vi "Bootloader.vi"() -> ()   [LabVIEW 2010]
uses:
  <vilib>/Utility/sysdir.llb/System Directory Type.ctl
  <vilib>/Instr/_visa.llb/VISA Configure Serial Port (Instr).vi
panel:
  in  "start path":path=path "<Not A Path>"
  in  "Run 3":bool
  in  "Run 2":bool
  in  "Exit":bool
  in  "Run":bool
  in  "Resource name:":refnum<visa-resource-name>
  in  "Path to firmware file (.hex):":path
  # "Caution: Make sure the right Firmware file is selected before Update the Harp device. Selecting\na Firmware that was not designed for the target Harp device may cause permanent damage."
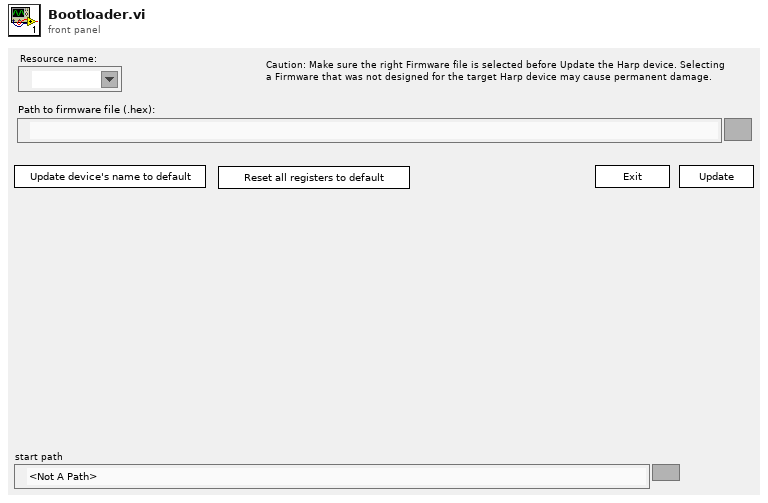
[diagram p1: front panel]
types:
  T1 = typedef "System Directory Type.ctl" = i32
  T2 = cluster{"reg. address":u8, "address content (en)":u8, "address content (dis)":u8, "fw .hex file path":path, "updater path":path}
  T3 = cluster{"reg. address":u8, "address content (en)":u8, "address content (dis)":u8, "Has .X":bool}[]
  T4 = cluster{"reg. address":u8, "address content (en)":u8, "address content (dis)":u8, "Has .X":bool}
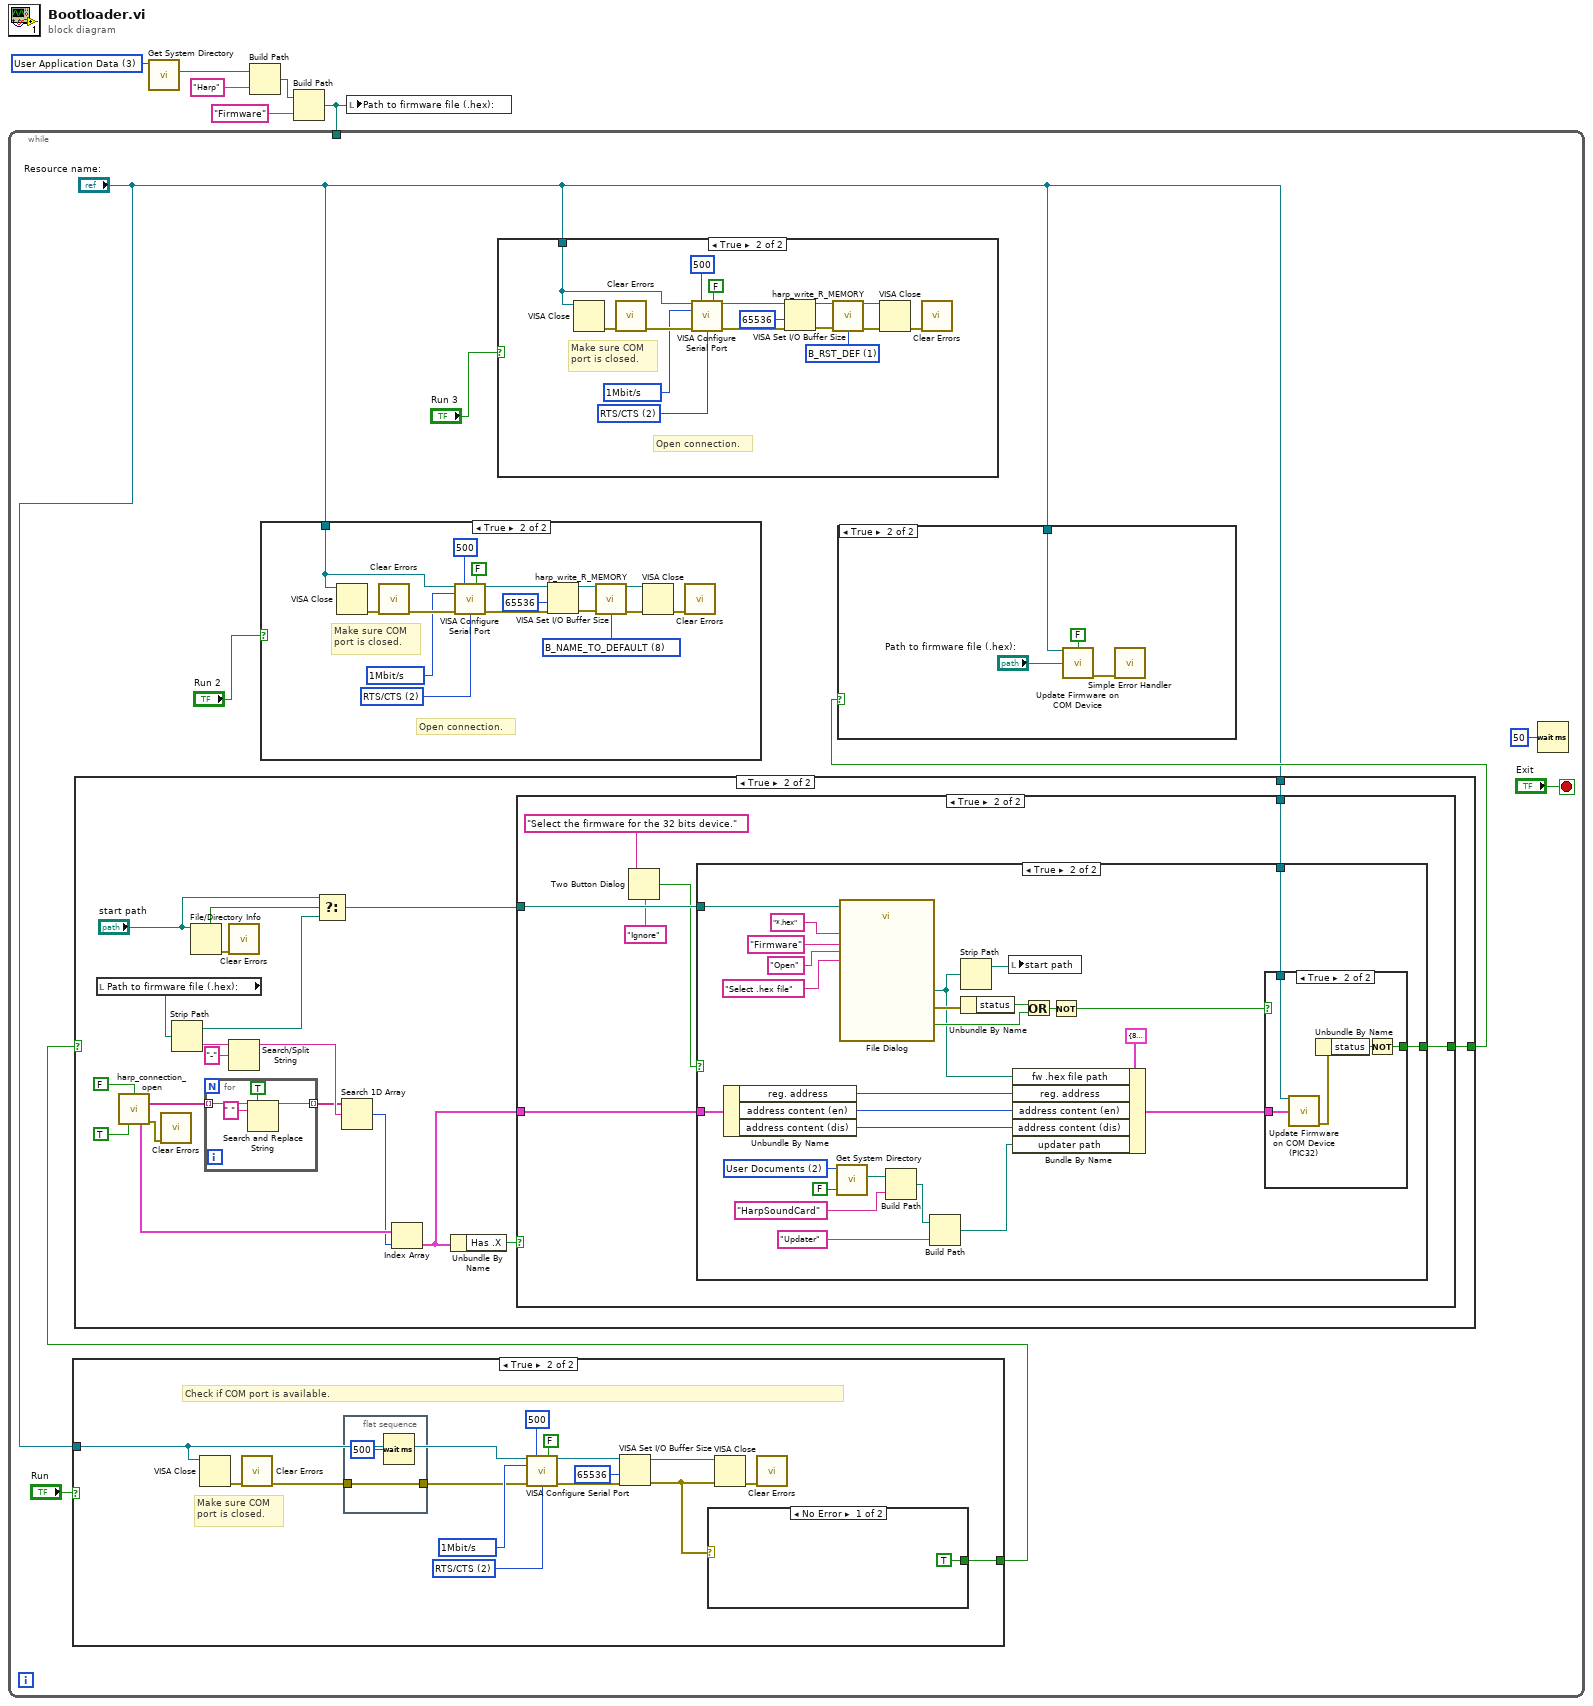
[diagram p0: block diagram]
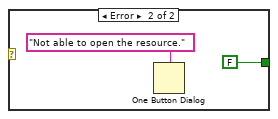
[diagram p3: hidden frame]
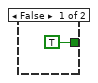
[diagram p5: hidden frame]
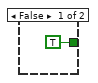
[diagram p6: hidden frame]
diagram:
  w4 = T1 3 items=["User Home"=0, "User Desktop"=1, "User Documents"=2, "User Application Data"=3, "User Preferences"=4, "User Temporary"=5, "Public Documents"=6, "Public Application Data"=7, "Public Preferences"=8, "Public Cache"=13, "System Core Libraries"=9, "System Installed Libraries"=10, "Application Files"=11, "Boot Volume Root"=12] ("system directory type")
  n1 = call <vilib>:"Get System Directory.vi"("system directory type"=w4) -> ("system directory"=w5:path)  [unwired: 10 in]
  n2 = Build Path(base path=w5, name or relative path="Harp") -> (appended path=w2:path)
  n3 = Build Path(base path=w2, name or relative path="Firmware") -> (appended path=w1:path)
  n4 = while {
    tunnel: w1 -> [_]
    stop <- "Exit" stop-if-true
    n5 = case shown="True" "Run" {
      selector: "Run" -> [w15 _]
      tunnel: "Resource name:" -> [_ w21]
      tunnel: [w15 w16] -> w7
      frame False {
      }
      frame True {
        w26 = u32 1000000 items=["250Kbit/s"=250000, "500kbit/s"=500000, "1Mbit/s"=1000000, "2Mbit/s"=2000000, "4Mbit/s"=4000000] ("baud rate")
        w27 = u16 2 items=["None", "XON/XOFF", "RTS/CTS", "XON/XOFF & RTS/CTS", "DTR/DSR", "XON/XOFF & DTR/DSR"] ("flow control (0:none)")
        # "Check if COM port is available."
        # "Make sure COM\nport is closed."
        n6 = VISA Close(VISA resource name=w21) -> (error out=w30:errorcluster)  [unwired: 1 in]
        n7 = call <vilib>:"Clear Errors.vi"("error in (no error)"=w30) -> ("error out"=w19:errorcluster)  [unwired: 6 in]
        n8 = flat-sequence {
          tunnel: w19 -> [w35]
          tunnel: [w35] -> w18
          frame #0 {
            n9 = Wait (ms)(milliseconds to wait=u32 500) -> ()  [unwired: 1 out]
          }
        }
        n10 = call-poly "VISA Configure Serial Port"("VISA resource name"=w21, "timeout (10sec)"=u32 500, "Enable Termination\nChar (T)"=FALSE ("Enable Termination\nChar (T)"), "baud rate (9600)"=w26, "error in (no error)"=w18, "flow control (0:none)"=w27) -> ("VISA resource name out"=w23:refnum<visa-resource-name>, "error out"=w24:errorcluster)  [unwired: 8 in]
        n11 = VISA Set I/O Buffer Size(VISA resource name=w23, size (4096)=u32 65536, error in (no error)=w24) -> (VISA resource name out=w20:refnum<visa-resource-name>, error out=w17:errorcluster)  [unwired: 1 in]
        n12 = case shown="No Error" w17 {
          tunnel: [TRUE FALSE] -> w16
          frame No Error {
          }
          frame Error {
            n13 = One Button Dialog(message="Not able to open the resource.") -> ()  [unwired: 1 in, 1 out]
          }
        }
        n14 = VISA Close(VISA resource name=w20, error in (no error)=w17) -> (error out=w22:errorcluster)
        n15 = call <vilib>:"Clear Errors.vi"("error in (no error)"=w22) -> ()  [unwired: 6 in, 1 out]
      }
    }
    n16 = case shown="True" w7 {
      selector: w7 -> [w36 _]
      tunnel: "Resource name:" -> [_ w40]
      tunnel: [w36 w39] -> w10
      frame False {
      }
      frame True {
        n17 = local read "Path to firmware file (.hex):"() -> (w44:path)
        n18 = call "harp_connection_open.vi"("launch dialog"=FALSE, "get lists only"=TRUE) -> ("Devices Name List"=w41:string[], "Devices X. settings"=w50:T3, "error out"=w42:errorcluster)  [unwired: 8 in, 3 out]
        n19 = call <vilib>:"Clear Errors.vi"("error in (no error)"=w42) -> ()  [unwired: 6 in, 1 out]
        n20 = Strip Path(path=w44) -> (stripped path=w54:path, name=w45:string)
        n21 = File/Directory Info(path="start path") -> (directory=w52:bool, error out=w37:errorcluster)  [unwired: 1 in, 5 out]
        n22 = for {
          tunnel: w41 -> [w101] mode=indexing
          tunnel: [w102] -> w47 mode=indexing
          n23 = Search and Replace String(replace all?=TRUE ("replace all? (F)"), input string=w101, search string=" ") -> (result string=w102:string)  [unwired: 5 in, 3 out]
        }
        n24 = call <vilib>:"Clear Errors.vi"("error in (no error)"=w37) -> ()  [unwired: 6 in, 1 out]
        n25 = Search/Split String(string=w45, search string/char (-)="-") -> (substring before match=w48:string)  [unwired: 1 in, 2 out]
        n26 = Select(t="start path", s=w52, f=w54) -> (s? t:f=w55:path)
        n27 = Search 1D Array(1D array=w47, element=w48) -> (index of element=w49:i32)  [unwired: 1 in]
        n28 = Index Array(array=w50, index=w49) -> (element=w51:T4)
        n29 = Unbundle By Name(w51) -> ("Has .X"=w56:bool)
        n30 = case shown="True" w56 {
          tunnel: w51 -> [_ w64]
          tunnel: w55 -> [_ w63]
          tunnel: w40 -> [_ w61]
          tunnel: [TRUE ("get lists only") w60] -> w39
          frame False {
          }
          frame True {
            n31 = Two Button Dialog(message="Select the firmware for the 32 bits device.", 1:"Ignore" ("F button name (\"Cancel\")")) -> (T button?=w58:bool)  [unwired: 1 in]
            n32 = case shown="True" w58 {
              tunnel: w64 -> [_ w92]
              tunnel: w63 -> [_ w91]
              tunnel: w61 -> [_ w90]
              tunnel: [TRUE w89] -> w60
              frame False {
              }
              frame True {
                w69 = T1 2 items=["User Home"=0, "User Desktop"=1, "User Documents"=2, "User Application Data"=3, "User Preferences"=4, "User Temporary"=5, "Public Documents"=6, "Public Application Data"=7, "Public Preferences"=8, "Public Cache"=13, "System Core Libraries"=9, "System Installed Libraries"=10, "Application Files"=11, "Boot Volume Root"=12] ("system directory type")
                n33 = Unbundle By Name(w92) -> ("reg. address"=w85:u8, "address content (en)"=w86:u8, "address content (dis)"=w87:u8)
                n34 = call <vilib>:"Get System Directory.vi"("create directory if not found? (F)"=FALSE, "system directory type"=w69) -> ("system directory"=w71:path)  [unwired: 9 in]
                n35 = call "File Dialog"("start path"=w91, "prompt"="Select .hex file" ("button label"), "button label"="Open", "pattern (all files)"="*.hex", "pattern label"="Firmware" ("button label")) -> ("selected path"=w76:path, "cancelled"=w77:bool, "error out"=w79:errorcluster)  [unwired: 7 in, 1 out]
                n36 = Build Path(base path=w71, name or relative path="HarpSoundCard") -> (appended path=w73:path)
                n37 = Build Path(base path=w73, name or relative path="Updater") -> (appended path=w68:path)
                n38 = Strip Path(path=w76) -> (stripped path=w80:path)  [unwired: 1 out]
                n39 = Unbundle By Name(w79) -> ("status"=w78:bool)
                n40 = local write "start path"(w80) -> ()
                n41 = Bundle By Name(cluster=T2 {"reg. address"=82, "address content (en)"=82, "address content (dis)"=82, "fw .hex file path"=path "Fir", "updater path"=path "Fir"} (".X settings"), "fw .hex file path"=w76, "reg. address"=w85, "address content (en)"=w86, "address content (dis)"=w87, "updater path"=w68) -> (w75:T2)
                n42 = Or(x=w78, y=w77) -> (x .or. y?=w67:bool)
                n43 = Not(x=w67) -> (.not. x?=w66:bool)
                n44 = case shown="True" w66 {
                  selector: w66 -> [w93 _]
                  tunnel: w75 -> [_ w98]
                  tunnel: w90 -> [_ w97]
                  tunnel: [w93 w94] -> w89
                  frame False {
                  }
                  frame True {
                    n45 = call "Update Firmware on COM Device (PIC32).vi"("VISA resource name"=w97, ".X settings"=w98) -> ("error out"=w96:errorcluster)  [unwired: 13 in]
                    n46 = Unbundle By Name(w96) -> ("status"=w95:bool)
                    n47 = Not(x=w95) -> (.not. x?=w94:bool)
                  }
                }
              }
            }
          }
        }
      }
    }
    n48 = case shown="True" "Run 2" {
      tunnel: "Resource name:" -> [_ w119]
      frame False {
      }
      frame True {
        w131 = u16 8 items=["B_RST_DEF"=1, "B_RST_EE"=2, "B_RST_SAVE"=4, "B_NAME_TO_DEFAULT"=8] ("reset mode")
        w124 = u32 1000000 items=["250Kbit/s"=250000, "500kbit/s"=500000, "1Mbit/s"=1000000, "2Mbit/s"=2000000, "4Mbit/s"=4000000] ("baud rate")
        w123 = u16 2 items=["None", "XON/XOFF", "RTS/CTS", "XON/XOFF & RTS/CTS", "DTR/DSR", "XON/XOFF & DTR/DSR"] ("flow control (0:none)")
        # "Open connection."
        # "Make sure COM\nport is closed."
        n49 = VISA Close(VISA resource name=w119) -> (error out=w120:errorcluster)  [unwired: 1 in]
        n50 = call <vilib>:"Clear Errors.vi"("error in (no error)"=w120) -> ("error out"=w127:errorcluster)  [unwired: 6 in]
        n51 = call-poly "VISA Configure Serial Port"("VISA resource name"=w119, "timeout (10sec)"=u32 500, "Enable Termination\nChar (T)"=FALSE ("Enable Termination\nChar (T)"), "baud rate (9600)"=w124, "error in (no error)"=w127, "flow control (0:none)"=w123) -> ("VISA resource name out"=w128:refnum<visa-resource-name>, "error out"=w126:errorcluster)  [unwired: 8 in]
        n52 = VISA Set I/O Buffer Size(VISA resource name=w128, size (4096)=u32 65536, error in (no error)=w126) -> (VISA resource name out=w130:refnum<visa-resource-name>, error out=w129:errorcluster)  [unwired: 1 in]
        n53 = call "harp_write_R_MEMORY.vi"("port"=w130, "error in (no error)"=w129, "reset mode"=w131) -> ("port out"=w133:refnum<visa-resource-name>, "error out"=w132:errorcluster)  [unwired: 11 in]
        n54 = VISA Close(VISA resource name=w133, error in (no error)=w132) -> (error out=w134:errorcluster)
        n55 = call <vilib>:"Clear Errors.vi"("error in (no error)"=w134) -> ()  [unwired: 6 in, 1 out]
      }
    }
    n56 = case shown="True" "Run 3" {
      tunnel: "Resource name:" -> [_ w103]
      frame False {
      }
      frame True {
        w115 = u16 1 items=["B_RST_DEF"=1, "B_RST_EE"=2, "B_RST_SAVE"=4, "B_NAME_TO_DEFAULT"=8] ("reset mode")
        w108 = u32 1000000 items=["250Kbit/s"=250000, "500kbit/s"=500000, "1Mbit/s"=1000000, "2Mbit/s"=2000000, "4Mbit/s"=4000000] ("baud rate")
        w107 = u16 2 items=["None", "XON/XOFF", "RTS/CTS", "XON/XOFF & RTS/CTS", "DTR/DSR", "XON/XOFF & DTR/DSR"] ("flow control (0:none)")
        # "Open connection."
        # "Make sure COM\nport is closed."
        n57 = VISA Close(VISA resource name=w103) -> (error out=w104:errorcluster)  [unwired: 1 in]
        n58 = call <vilib>:"Clear Errors.vi"("error in (no error)"=w104) -> ("error out"=w111:errorcluster)  [unwired: 6 in]
        n59 = call-poly "VISA Configure Serial Port"("VISA resource name"=w103, "timeout (10sec)"=u32 500, "Enable Termination\nChar (T)"=FALSE ("Enable Termination\nChar (T)"), "baud rate (9600)"=w108, "error in (no error)"=w111, "flow control (0:none)"=w107) -> ("VISA resource name out"=w112:refnum<visa-resource-name>, "error out"=w110:errorcluster)  [unwired: 8 in]
        n60 = VISA Set I/O Buffer Size(VISA resource name=w112, size (4096)=u32 65536, error in (no error)=w110) -> (VISA resource name out=w114:refnum<visa-resource-name>, error out=w113:errorcluster)  [unwired: 1 in]
        n61 = call "harp_write_R_MEMORY.vi"("port"=w114, "error in (no error)"=w113, "reset mode"=w115) -> ("port out"=w117:refnum<visa-resource-name>, "error out"=w116:errorcluster)  [unwired: 11 in]
        n62 = VISA Close(VISA resource name=w117, error in (no error)=w116) -> (error out=w118:errorcluster)
        n63 = call <vilib>:"Clear Errors.vi"("error in (no error)"=w118) -> ()  [unwired: 6 in, 1 out]
      }
    }
    n64 = case shown="True" w10 {
      tunnel: "Resource name:" -> [_ w135]
      frame False {
      }
      frame True {
        n65 = call "Update Firmware on COM Device.vi"("VISA resource name"=w135, "Skip Bootloader call"=FALSE, ".hex path"="Path to firmware file (.hex):") -> ("error out"=w136:errorcluster)  [unwired: 12 in]
        n66 = call <vilib>:"Simple Error Handler.vi"("error in (no error)"=w136) -> ()  [unwired: 4 in, 5 out]
      }
    }
    n67 = Wait (ms)(milliseconds to wait=u32 50) -> ()  [unwired: 1 out]
  }
  n68 = local write "Path to firmware file (.hex):"(w1) -> ()
